vi "Test Overrides Has Mock Class on Dynamic Connectors.vi"(8 "error in (no error)":errorcluster, 11 "Test Case In":refnum<class "Mock Class Generator Test.lvclass">) -> (0 "error out":errorcluster, 3 "Test Case Out":refnum<class "Mock Class Generator Test.lvclass">)   [LabVIEW 2020, in "Mock Class Generator Test.lvclass"]
uses:
  Mock Class Generator Test.lvclass
  C:/Program Files (x86)/National Instruments/LabVIEW 2020/vi.lib/Astemes/LUnit/Test Case.lvclass
  <vilib>/Astemes/LUnit/Test Case.lvclass/Test Case.ctl
  <vilib>/Astemes/LUnit/Append Pass Result.vi
  <vilib>/Astemes/LUnit/Append Fail Result.vi
  Mock Class Generator Test.lvclass/Mock Class Generator Test.ctl
  source/Mock Class Generator/Mock Class Generator.lvclass
  <vilib>/Astemes/LUnit/Test Case.lvclass
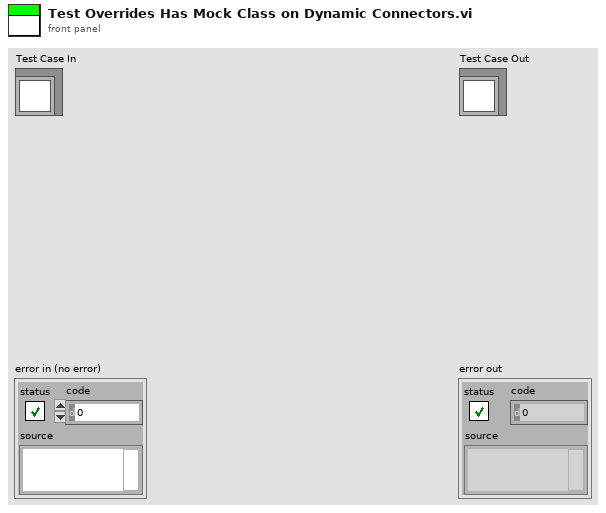
[diagram p1: front panel]
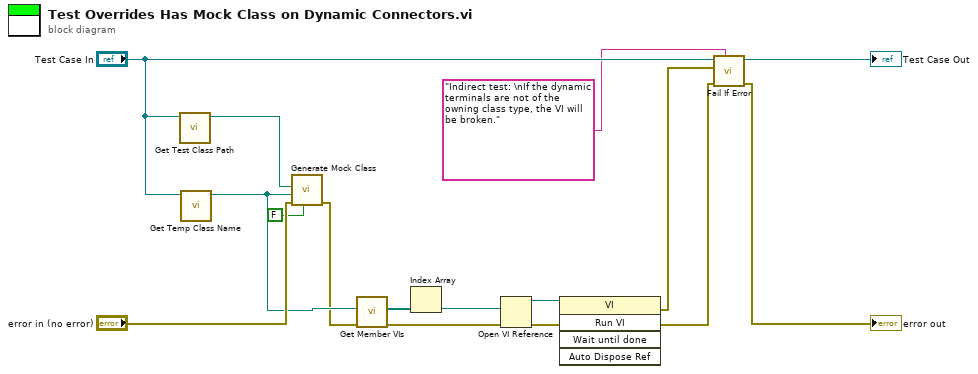
[diagram p0: block diagram]
diagram:
  n1 = call "Get Test Class Path.vi"("Mock Class Generator Test in"="Test Case In") -> ("Test Class Path"=w11:path)  [unwired: 10 in]
  n2 = call "Get Temp Class Name.vi"("Mock Class Generator Test in"="Test Case In") -> ("Test Class Path"=w10:path)  [unwired: 10 in]
  n3 = call "Generate Mock Class.vi"("Add to lvproj?"=FALSE, "error in (no error)"="error in (no error)", "Destination Class Path"=w10, "Source Class Path"=w11) -> ("error out"=w9:errorcluster)  [unwired: 7 in]
  n4 = call "Get Member VIs.vi"("error in (no error)"=w9, "Test Class Path"=w10) -> ("error out"=w8:errorcluster, "Array"=w7:path[])  [unwired: 8 in]
  n5 = Index Array(array=w7) -> (element=w5:path)  [unwired: 1 in]
  n6 = Open VI Reference(vi path=w5, error in (no error)=w8) -> (vi reference=w4:refnum<vi>, error out=w6:errorcluster)  [unwired: 4 in]
  n7 = invoke class="VI" method="Run VI"(reference=w4) -> (error out=w3:errorcluster)  [unwired: 4 in, 4 out]
  n8 = call <vilib>:"Fail If Error.vi"("Description"="Indirect test: \nIf the dynamic terminals are not of the owning class type, the VI will be broken.", "error in (no error)"=w6, "Assert error"=w3, "LUnit Test Case In"="Test Case In") -> ("error out"=→"error out":errorcluster, "LUnit Test Case Out"=→"Test Case Out":refnum<class "Mock Class Generator Test.lvclass">)  [unwired: 6 in]
